vi "PH_Sequencer_Watch.PC _BooleanState.vi"(0 "i ref in":refnum<vi>, 2 "serviceName":string, 3 "Status":T1 items=["no info", "off/false/out", "on/true/in", "Failure", "Alarm", "Status 1", "Status 2", "Status 3"], 5 "error IO":errorcluster) -> (14 "i ref out":refnum<vi>, 19 "error out":errorcluster)   [LabVIEW 2014, in "PH_Sequencer_Watch.lvlib"]
doc: "This VI sets incoming values to the GUI element."
uses:
  PH_Sequencer_Watch.lvlib
  PH_StatusHandler/PH_StatusHandler.Status.ctl
  PH_Common/PH_Common.lvlib
  PH_StatusHandler/PH_StatusHandler.lvlib
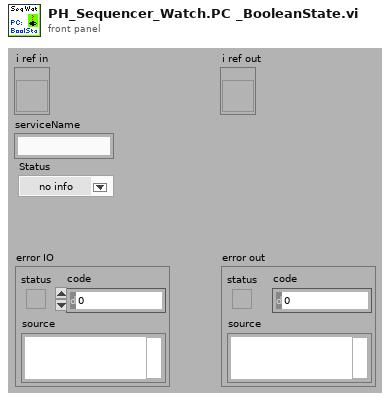
[diagram p1: front panel]
types:
  T1 = typedef "PH_StatusHandler.lvlib/PH_StatusHandler.Status.ctl" = i16
  T2 = typedef "PH_Sequencer_Watch.lvlib/PH_Sequencer_Watch.i attribute.ctl" = cluster{"GUI Refs":cluster{"Shot ID":refnum<vi>, "Sequencer SM State":refnum<vi>, "Remaining Time":refnum<vi>, "PHELIX_Timing_T2":refnum<vi>, "T2-Unit-Dummy":refnum<vi>, "fs_Synchrolock_Watch":refnum<vi>, "Experiment_Vacuum_Control_Experiment":refnum<vi>}, "Status Synchrolock":T1, "Exp - Pressure":dbl, "Exp - Limit":dbl, "Heads":T3[], "Refs BooleanState":refnum<vi>[]}
  T3 = typedef "PH_Sequencer_Watch.lvlib/PH_Sequencer_Watch.Head Information.ctl" = cluster{"Ref Volt":refnum<vi>, "PU":T4}
  T4 = typedef "PH_PP_Common.lvlib/PH_PP_Common.PUs.ctl" = enum16{"no Info", "PA-19mm-1", "PA-19mm-2", "PA-45mm-PILC", "PA-45mm-MAIN", "MA-PU-1", "MA-PU-2", "MA-PU-3", "MA-PU-4", "MA-PU-5", "MA-PU-6", "MA-FR", "MA-PILC", "PA-45mm-DP"}
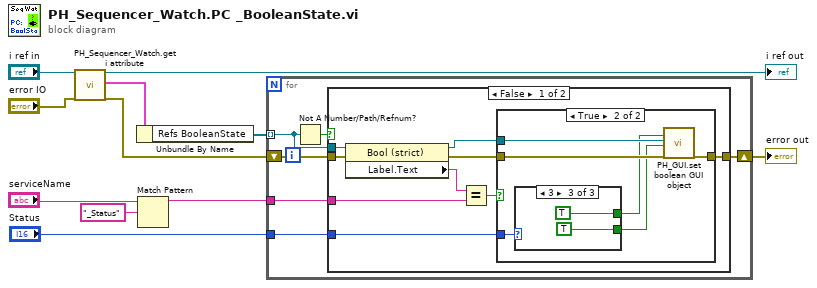
[diagram p0: block diagram]
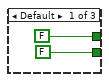
[diagram p3: hidden frame]
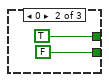
[diagram p4: hidden frame]
diagram:
  n1 = call "PH_Sequencer_Watch.get i attribute.vi"("i ref in"="i ref in", "error in (no error)"="error IO") -> ("i ref out"=→"i ref out":refnum<vi>, "i attribute"=w7:T2, "error out"=w6:errorcluster)  [unwired: 15 in]
  n2 = Unbundle By Name(w7) -> ("Refs BooleanState"=w8:refnum<vi>[])
  n3 = Match Pattern(string="serviceName", regular expression="_Status") -> (before substring=w2:string)  [unwired: 1 in, 3 out]
  n4 = for {
    tunnel: w8 -> [w16] mode=indexing
    shift-right: [w15] -> w5
    shift-left: w6 -> [w14]
    tunnel: w2 -> [w13]
    tunnel: "Status" -> [w12]
    n5 = Not A Number/Path/Refnum?(number/path/refnum=w16) -> (NaN/Path/Refnum?=w17:bool)
    n6 = case shown="False" w17 {
      tunnel: w16 -> [w26 _]
      tunnel: [w22 w40] -> w15
      tunnel: w14 -> [w25 w40]
      tunnel: w13 -> [w19 _]
      tunnel: w12 -> [w20 _]
      frame False {
        n7 = property class="Bool (strict)"(reference=w26, error in=w25) -> (reference out=w21:refnum<vi>, error out=w23:errorcluster, "Label.Text"=w24:string)
        n8 = Equal?(x=w24, y=w19) -> (x = y?=w18:bool)
        n9 = case shown="True" w18 {
          tunnel: w23 -> [w27 w33]
          tunnel: [w27 w32] -> w22
          tunnel: w21 -> [_ w31]
          tunnel: w20 -> [_ w30]
          frame False {
          }
          frame True {
            n10 = case shown="3" w30 {
              tunnel: [FALSE TRUE TRUE] -> w29
              tunnel: [FALSE FALSE TRUE] -> w28
              frame Default {
              }
              frame 0 {
              }
              frame 3 {
              }
            }
            n11 = call "PH_GUI.set boolean GUI object.vi"("Visible (true)"=w29, "Boolean Knob GUI Ref"=w31, "Value"=w28, "error in (no error)"=w33) -> ("error out"=w32:errorcluster)  [unwired: 15 in]
          }
        }
      }
      frame True {
      }
    }
  }
  "error out" <- w5
